vi "FeedbackDecode_WriteEyeParams.vi"(6 "FileTime":string, 7 "DataPath":path=path "D:/FeedbackDecode/00000000-000000", 8 "ErrorIn":errorcluster, 9 "PupilClust":T1, 11 "Mode":enum16{"Initialize", "Run", "Close"}(ring)) -> (0 "ErrorOut":errorcluster, 2 "EyeParamsName":path)   [LabVIEW 2020]
uses:
  FeedbackDecode_Globals.vi
panel:
  out "EyeParamsFID":refnum<file>
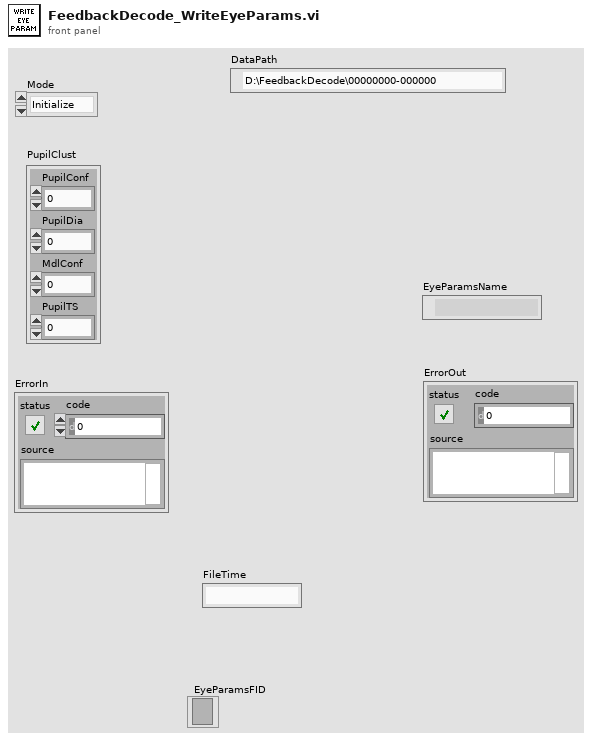
[diagram p1: front panel]
types:
  T1 = cluster{"PupilConf":dbl, "PupilDia":dbl, "MdlConf":dbl, "PupilTS":dbl}
  T2 = enum16{"open", "replace", "create", "open or create", "replace or create", "replace or create with confirmation"}
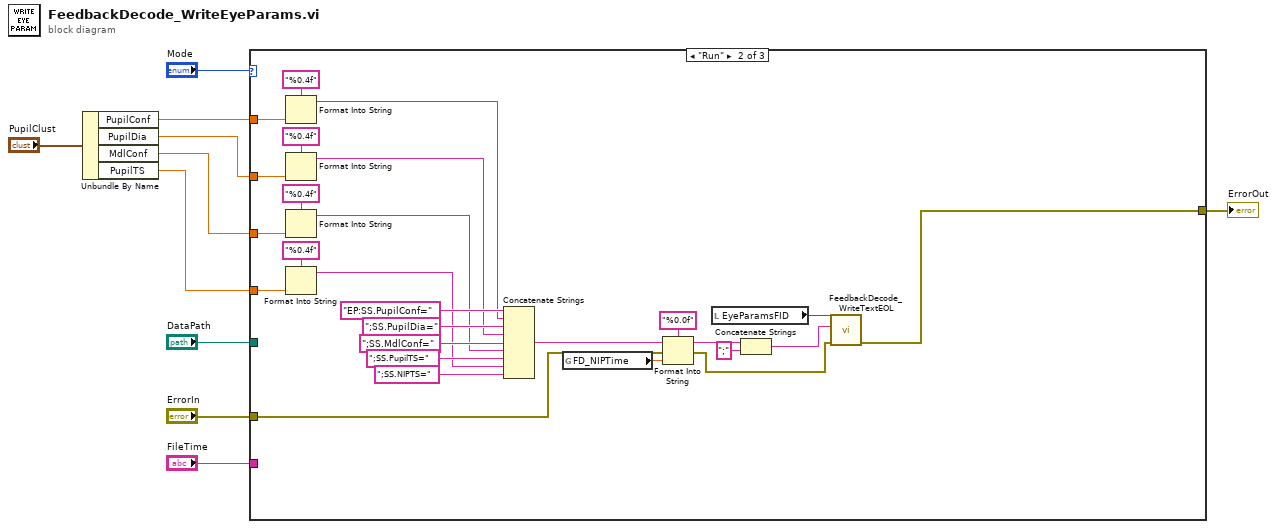
[diagram p0: block diagram]
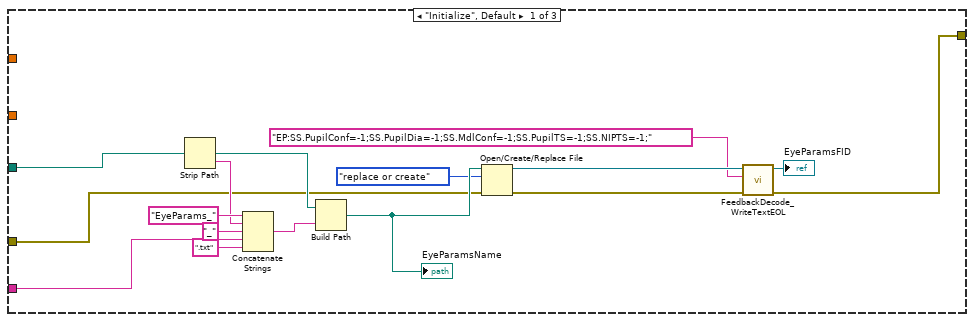
[diagram p2: hidden frame]
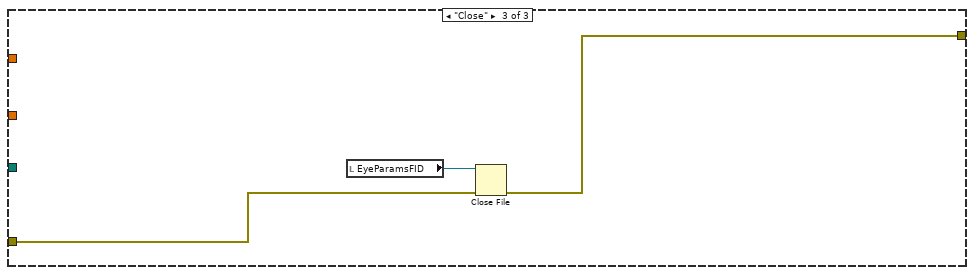
[diagram p3: hidden frame]
diagram:
  n1 = Unbundle By Name("PupilClust") -> ("PupilConf"=w5:dbl, "PupilDia"=w4:dbl, "MdlConf"=w3:dbl, "PupilTS"=w1:dbl)
  n2 = case shown="\"Run\"" "Mode" {
    tunnel: "ErrorIn" -> [w15 w43 w55]
    tunnel: [w18 w44 w54] -> w8
    tunnel: "DataPath" -> [w16 _ _]
    tunnel: "FileTime" -> [w12 _ _]
    tunnel: w5 -> [_ w40 _]
    tunnel: w4 -> [_ w38 _]
    tunnel: w3 -> [_ w33 _]
    tunnel: w1 -> [_ w30 _]
    frame "Initialize", Default {
      n3 = Strip Path(path=w16) -> (name=w20:string)  [unwired: 1 out]
      n4 = Concatenate Strings("EyeParams_" ("name or relative path"), w20, "_" ("string"), w12, ".txt" ("string")) -> (w21:string)
      n5 = Build Path(base path=w16, name or relative path=w21) -> (appended path=w25:path)
      "EyeParamsName" <- w25
      n6 = Open/Create/Replace File(file path (use dialog)=w25, error in=w15, operation (0:open)=T2."replace or create") -> (refnum out=w19:refnum<file>, error out=w13:errorcluster)  [unwired: 3 in, 1 out]
      n7 = call "FeedbackDecode_WriteTextEOL.vi"("error in"=w13, "text"="EP:SS.PupilConf=-1;SS.PupilDia=-1;SS.MdlConf=-1;SS.PupilTS=-1;SS.NIPTS=-1;" ("string"), "refnum in"=w19) -> ("error out"=w18:errorcluster, "refnum out"=→"EyeParamsFID":refnum<file>)  [unwired: 7 in]
    }
    frame "Run" {
      n8 = Format Into String(format string="%0.4f", w40) -> (resulting string=w37:string)  [unwired: 2 in, 1 out]
      n9 = Format Into String(format string="%0.4f", w38) -> (resulting string=w35:string)  [unwired: 2 in, 1 out]
      n10 = Format Into String(format string="%0.4f", w33) -> (resulting string=w27:string)  [unwired: 2 in, 1 out]
      n11 = Format Into String(format string="%0.4f", w30) -> (resulting string=w26:string)  [unwired: 2 in, 1 out]
      n12 = Concatenate Strings("EP:SS.PupilConf=" ("string"), w37, ";SS.PupilDia=" ("string"), w35, ";SS.MdlConf=" ("string"), w27, ";SS.PupilTS=" ("string"), w26, ";SS.NIPTS=" ("string")) -> (w47:string)
      n13 = global read "FeedbackDecode_Globals.vi" "FD_NIPTime"() -> (w42:dbl)
      n14 = Format Into String(format string="%0.0f", initial string=w47, error in=w43, w42) -> (resulting string=w49:string, error out=w45:errorcluster)
      n15 = local read "EyeParamsFID"() -> (w52:refnum<file>)
      n16 = Concatenate Strings(w49, ";" ("string")) -> (w46:string)
      n17 = call "FeedbackDecode_WriteTextEOL.vi"("error in"=w45, "text"=w46, "refnum in"=w52) -> ("error out"=w44:errorcluster)  [unwired: 7 in, 1 out]
    }
    frame "Close" {
      n18 = local read "EyeParamsFID"() -> (w53:refnum<file>)
      n19 = Close File(refnum=w53, error in=w55) -> (error out=w54:errorcluster)  [unwired: 1 out]
    }
  }
  "ErrorOut" <- w8
